vi "Find and Call MeasurementLink Plugin.vi"() -> ()   [LabVIEW 2020]
uses:
  <vilib>/MeasurementLink/MeasurementLink Discovery Client/RPC Messages/ni_measurementlink_discovery_v1_ServiceLocation.ctl
  Measurement Configuration.ctl
  <vilib>/MeasurementLink/MeasurementLink Discovery Client/RPC Messages/ni_measurementlink_discovery_v1_EnumerateServicesRequest.ctl
  <vilib>/MeasurementLink/MeasurementLink Discovery Client/RPC Messages/ni_measurementlink_discovery_v1_ResolveServiceRequest.ctl
  Measurement Results.ctl
  Measurement Service Client V2/RPC Messages/ni_measurementlink_measurement_v2_MeasureRequest.ctl
  Measurement Service Client V2/RPC Messages/google_protobuf_Any.ctl
  Measurement Service Client V2/RPC Messages/ni_measurementlink_PinMapContext.ctl
  045899de-a912-426a-8a5d-a949b9672173.vi
  <vilib>/gRPC/LabVIEW gRPC Library/Server API/Translate Protobuf Error.vi
  <vilib>/AdvancedString/1D String Array to Delimited String.vi
  <vilib>/gRPC/LabVIEW gRPC Library/Server API/Server/Get Server DLL Path.vi
  <vilib>/MeasurementLink/MeasurementLink Discovery Client/MeasurementLink Discovery Client.lvlib
  <vilib>/gRPC/LabVIEW gRPC Library/grpc-lvsupport-release.lvlib
  Measurement Service Client V2/Measurement Service Client V2.lvlib
panel:
  in  "stop":bool
  out "waveform graph":dbl[](graph)
  out "available services":string[](array[string])
  in  "measurement configuration":T1={"Frequency"=1.0, "Amplitude"=1.0}
  out "error out":errorcluster
  out "matched service":T2
  out "Found?":bool
  in  "address":string="localhost:42000"
  in  "service to run":string="GetSineSignal_LabVIEW"
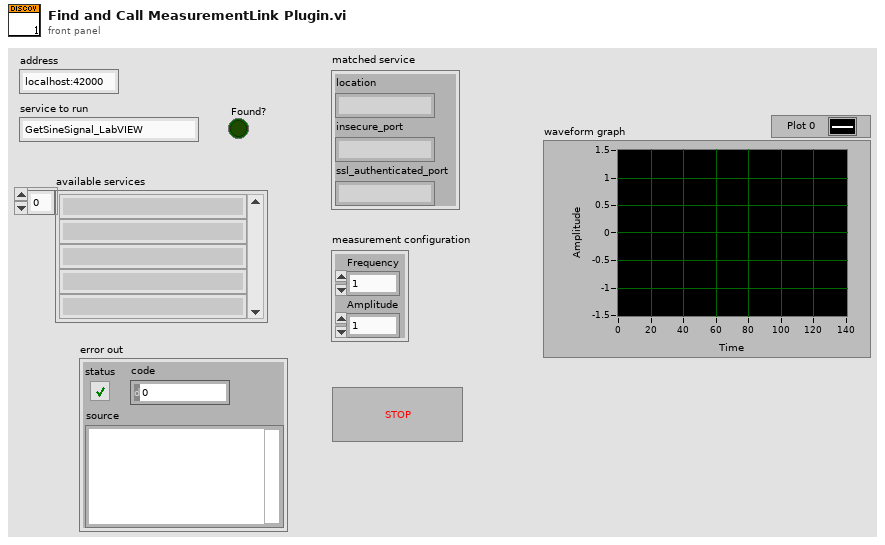
[diagram p1: front panel]
types:
  T1 = typedef "Measurement Configuration.ctl" = cluster{"Frequency":dbl, "Amplitude":dbl}
  T2 = typedef "MeasurementLink Discovery Client.lvlib/ni_measurementlink_discovery_v1_ServiceLocation.ctl" = cluster{"location":string, "insecure_port":string, "ssl_authenticated_port":string}
  T3 = typedef "Measurement Results.ctl" = cluster{"Array":dbl[]}
  T4 = typedef "MeasurementLink Discovery Client.lvlib/ni_measurementlink_discovery_v1_ResolveServiceRequest.ctl" = cluster{"provided_interface":string, "service_class":string}
  T5 = typedef "MeasurementLink Discovery Client.lvlib/ni_measurementlink_discovery_v1_EnumerateServicesRequest.ctl" = cluster{"provided_interface":string}
  T6 = typedef "grpc-lvsupport-release.lvlib/grpcId.ctl" = u64
  T7 = typedef "MeasurementLink Discovery Client.lvlib/ni_measurementlink_discovery_v1_EnumerateServicesResponse.ctl" = cluster{"available_services":T8[]}
  T8 = typedef "MeasurementLink Discovery Client.lvlib/ni_measurementlink_discovery_v1_ServiceDescriptor.ctl" = cluster{"display_name":string, "description_url":string, "provided_interfaces":string[], "service_class":string, "annotations":T9[]}
  T9 = typedef "MeasurementLink Discovery Client.lvlib/ni_measurementlink_discovery_v1_ServiceDescriptor_AnnotationsEntry.ctl" = cluster{"key":string, "value":string}
  T10 = typedef "grpc-lvsupport-release.lvlib/Message Metadata.ctl" = cluster{"Version":i32, "Name":string, "Type Url":string, "Elements":T11[], "Has Oneof":bool}
  T11 = typedef "grpc-lvsupport-release.lvlib/Message Element Metadata.ctl" = cluster{"Field Name":string, "Embedded Message Name":string, "Protobuf Index":i32, "MessageElementType":T12, "Repeated":bool, "Is in Oneof":bool, "Oneof Container Name":string}
  T12 = typedef "grpc-lvsupport-release.lvlib/Message Element Type.ctl" = enum32{"Int32Value", "FloatValue", "DoubleValue", "BoolValue", "StringValue", "MessageValue", "Int64Value", "UInt32Value", "UInt64Value", "EnumValue", "Bytes", "Fixed64", "Fixed32", "SFixed64", "SFixed32", "SInt64", "SInt32"}
  T13 = typedef "Measurement Service Client V2.lvlib/ni_measurementlink_measurement_v2_MeasureRequest.ctl" = cluster{"configuration_parameters":T14, "pin_map_context":T15}
  T14 = typedef "Measurement Service Client V2.lvlib/google_protobuf_Any.ctl" = cluster{"type_url":string, "value":u8[]}
  T15 = typedef "Measurement Service Client V2.lvlib/ni_measurementlink_PinMapContext.ctl" = cluster{"pin_map_id":string, "sites":i32[]}
  T16 = typedef "grpc-lvsupport-release.lvlib/Any.ctl" = cluster{"Type Url":string, "Bytes":u8[]}
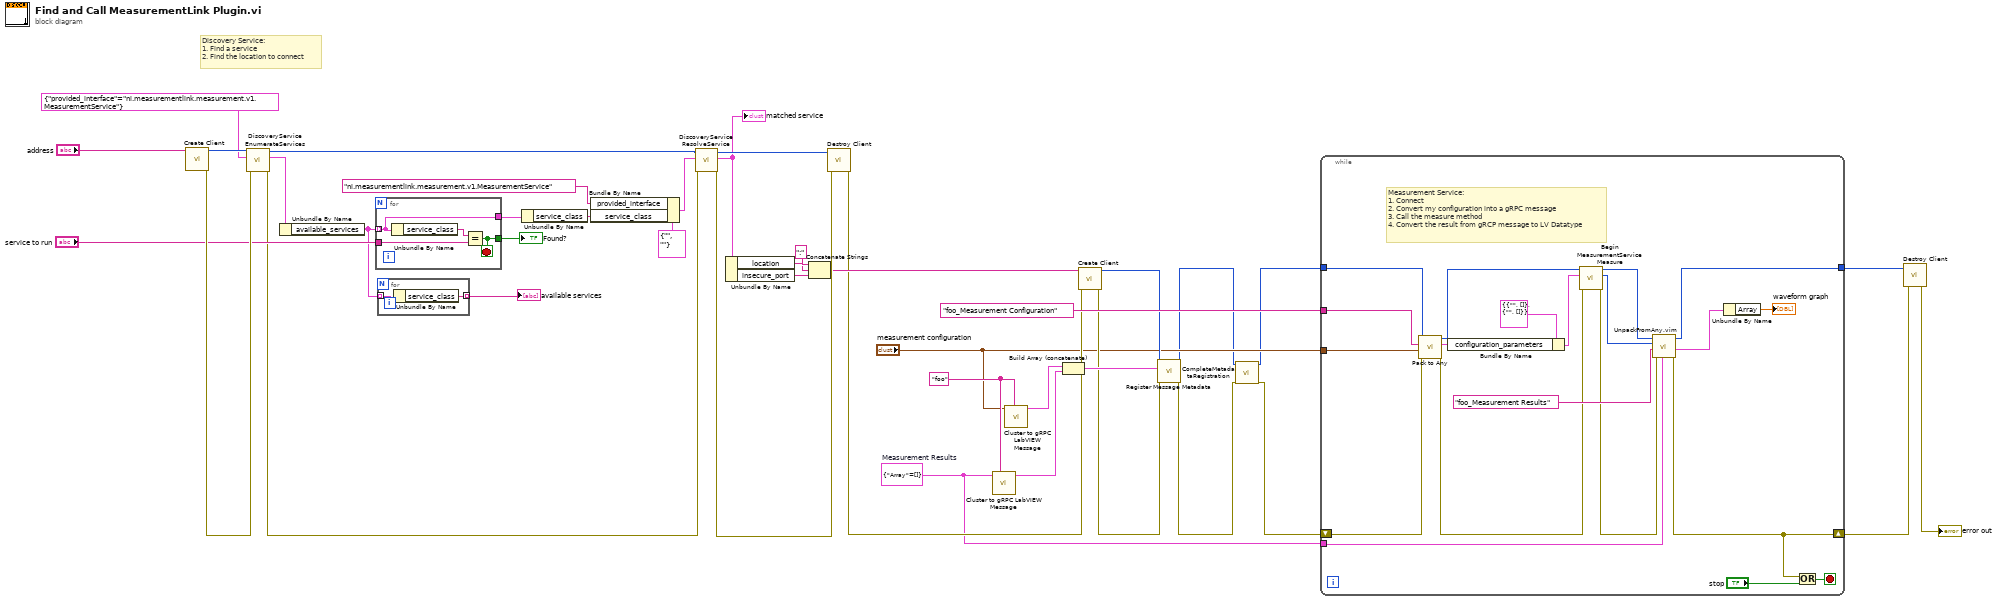
[diagram p0: block diagram]
diagram:
  w7 = T3 {"Array"=[]}  # Measurement Results
  w18 = "foo" ("Package Name")
  # "Discovery Service:\n1. Find a service\n2. Find the location to connect"
  n1 = call <vilib>:"Create Client.vi"("address"="address") -> ("error out"=w38:errorcluster, "gRPC ID Out"=w39:T6)  [unwired: 9 in]
  n2 = call <vilib>:"DiscoveryService EnumerateServices.vi"("error in"=w38, "Request Data"=T5 {"provided_interface"="ni.measurementlink.measurement.v1.MeasurementService"}, "gRPC ID"=w39) -> ("error out"=w31:errorcluster, "Response Data"=w36:T7, "gRPC ID out"=w32:T6)  [unwired: 6 in]
  n3 = Unbundle By Name(w36) -> ("available_services"=w17:T8[])
  n4 = for {
    tunnel: w17 -> [w42] mode=indexing
    tunnel: "service to run" -> [w43]
    tunnel: [w42] -> w33
    tunnel: [w41] -> w34
    stop <- w41 stop-if-true
    n5 = Unbundle By Name(w42) -> ("service_class"=w44:string)
    n6 = Equal?(x=w44, y=w43) -> (x = y?=w41:bool)
  }
  "Found?" <- w34
  n7 = for {
    tunnel: w17 -> [w46] mode=indexing
    tunnel: [w45] -> w16 mode=indexing
    n8 = Unbundle By Name(w46) -> ("service_class"=w45:string)
  }
  "available services" <- w16
  n9 = Unbundle By Name(w33) -> ("service_class"=w27:string)
  n10 = Bundle By Name(cluster=T4 {"provided_interface"="", "service_class"=""} ("Request Data"), "provided_interface"="ni.measurementlink.measurement.v1.MeasurementService", "service_class"=w27) -> (w25:T4)
  n11 = call <vilib>:"DiscoveryService ResolveService.vi"("error in"=w31, "Request Data"=w25, "gRPC ID"=w32) -> ("error out"=w30:errorcluster, "Response Data"=w24:T2, "gRPC ID out"=w29:T6)  [unwired: 6 in]
  "matched service" <- w24
  n12 = Unbundle By Name(w24) -> ("location"=w23:string, "insecure_port"=w21:string)
  n13 = Concatenate Strings(w23, ":" ("string"), w21) -> (w13:string)
  n14 = call <vilib>:"Destroy Client.vi"("error in"=w30, "gRPC ID"=w29) -> ("error out"=w12:errorcluster)  [unwired: 9 in]
  n15 = call <vilib>:"Cluster to gRPC LabVIEW Message.vi"("Package Name"=w18, "Cluster"=w7) -> ("gRPC Message Metadata []"=w19:T10[])  [unwired: 7 in, 2 out]
  n16 = call <vilib>:"Cluster to gRPC LabVIEW Message.vi"("Package Name"=w18, "Cluster"="measurement configuration") -> ("gRPC Message Metadata []"=w20:T10[])  [unwired: 7 in, 2 out]
  n17 = Build Array (concatenate)(w20, w19) -> (w15:T10[])
  n18 = call <vilib>:"Create Client.vi"("error in"=w12, "address"=w13) -> ("error out"=w11:errorcluster, "gRPC ID Out"=w10:T6)  [unwired: 8 in]
  n19 = call <vilib>:"Register Message Metadata.vi"("error in"=w11, "Messages"=w15, "gRPCid in"=w10) -> ("error out"=w3:errorcluster, "gRPCid out"=w5:T6)  [unwired: 7 in]
  n20 = call <vilib>:"CompleteMetadataRegistration.vi"("error in"=w3, "gRPC ID in"=w5) -> ("error out"=w2:errorcluster, "gRPC ID Out"=w4:T6)  [unwired: 8 in]
  n21 = while {
    tunnel: w4 -> [w52]
    tunnel: "foo_Measurement Configuration" ("Message Type") -> [w49]
    tunnel: [w47] -> w1
    tunnel: "measurement configuration" -> [w48]
    shift-right: [w53] -> w9
    shift-left: w2 -> [w65]
    tunnel: w7 -> [w56]
    stop <- w54 stop-if-true
    # "Measurement Service:\n1. Connect\n2. Convert my configuration into a gRPC message\n3. Call the measure method\n4. Convert the result from gRCP message to LV Datatype"
    n22 = call "Pack to Any.vi"("error in"=w65, "data to pack"=w48, "message type"=w49, "gRPC ID in"=w52) -> ("error out"=w51:errorcluster, "any"=w50:T16, "gRPC ID out"=w64:T6)  [unwired: 5 in]
    n23 = Bundle By Name(cluster=T13 {"configuration_parameters"={"type_url"="", "value"=[]}, "pin_map_context"={"pin_map_id"="", "sites"=[]}} ("Request Data"), "configuration_parameters"=w50) -> (w60:T13)
    n24 = call "Begin MeasurementService Measure.vi"("error in"=w51, "Request Data"=w60, "gRPC ID"=w64) -> ("error out"=w62:errorcluster, "Call Id Out"=w55:T6, "gRPC ID out"=w63:T6)  [unwired: 6 in]
    n25 = call "UnpackFromAny.vim"("Data Type"=w56, "error in"=w62, "Message Type"="foo_Measurement Results", "Any"=w55, "gRPCid in"=w63) -> ("error out"=w53:errorcluster, "Unpacked Value"=w57:T3, "gRPCid out"=w47:u64)  [unwired: 4 in]
    n26 = Unbundle By Name(w57) -> ("Array"=→"waveform graph":dbl[])
    n27 = Or(x=w53, y="stop") -> (x .or. y?=w54:bool)
  }
  n28 = call <vilib>:"Destroy Client.vi"("error in"=w9, "gRPC ID"=w1) -> ("error out"=→"error out":errorcluster)  [unwired: 9 in]
